vi "www template read file.vi"(6 "User Information":T1, 7 "HTTP Header (\"\")":string, 8 "error in (no error)":errorcluster, 11 "Template File (\"\")":string) -> (0 "error out":errorcluster, 3 "Page HTML":string, 5 "new HTTP Header":string)   [LabVIEW 2011]
uses:
  server/database/Users/User Record.ctl
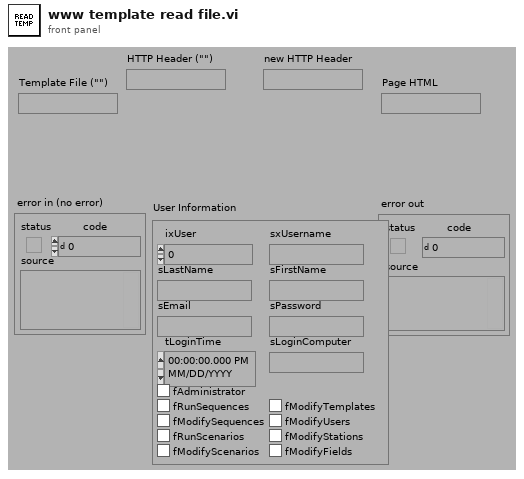
[diagram p1: front panel]
types:
  T1 = typedef "User Record.ctl" = cluster{"ixUser":i32, "sxUsername":string, "sLastName":string, "sFirstName":string, "sEmail":string, "sPassword":string, "tLoginTime":timestamp, "sLoginComputer":string, "fAdministrator":bool, "fRunSequences":bool, "fModifySequences":bool, "fRunScenarios":bool, "fModifyScenarios":bool, "fModifyTemplates":bool, "fModifyUsers":bool, "fModifyStations":bool, "fModifyFields":bool}
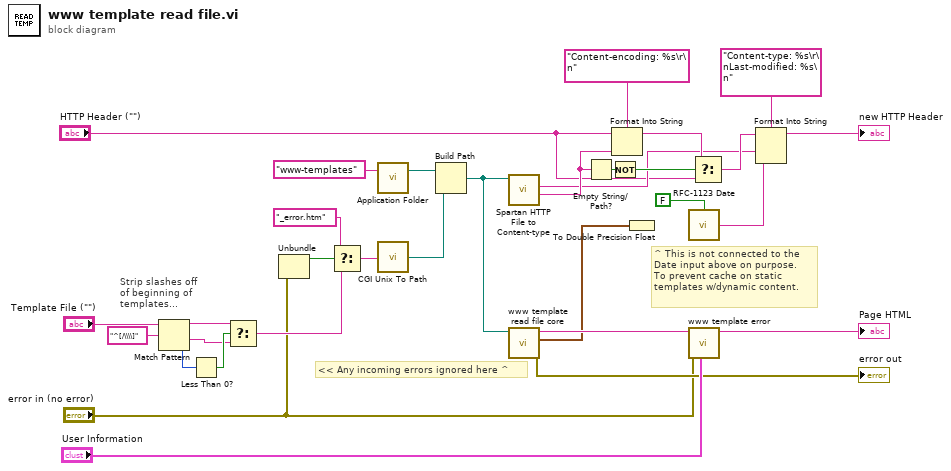
[diagram p0: block diagram]
diagram:
  # "Strip slashes off\nof beginning of\ntemplates..."
  # "^ This is not connected to the\nDate input above on purpose.\nTo prevent cache on static\ntemplates w/dynamic content."
  # "<< Any incoming errors ignored here ^"
  n1 = Match Pattern(string="Template File (\"\")", regular expression="^[/\\\\]") -> (before substring=w18:string, after substring=w17:string, offset past match=w20:i32)  [unwired: 2 out]
  n2 = Less Than 0?(x=w20) -> (x < 0?=w19:bool)
  n3 = Select(t=w18, s=w19, f=w17) -> (s? t:f=w9:string)
  n4 = Unbundle("error in (no error)") -> ("status"=w12:bool)  [unwired: 2 out]
  n5 = Select(t="_error.htm" ("format string"), s=w12, f=w9) -> (s? t:f=w10:string)
  n6 = call "Application Folder.vi"("Relative Path (\"\" - Folder)"="www-templates" ("name or relative path")) -> ("Application Folder"=w1:path)  [unwired: 2 in]
  n7 = call "CGI Unix To Path.vi"("unix path"=w10) -> ("platform path"=w22:path)  [unwired: 1 out]
  n8 = Build Path(base path=w1, name or relative path=w22) -> (appended path=w5:path)
  n9 = call "Spartan HTTP File to Content-type.vi"("file path"=w5) -> ("content-encoding"=w24:string, "content-type"=w23:string)  [unwired: 3 in, 6 out]
  n10 = call "www template read file core.vi"("Path"=w5) -> ("error out"=→"error out":errorcluster, "File Modified"=w3:timestamp, "File Content"=w6:string)  [unwired: 1 in, 7 out]
  n11 = Empty String/Path?(string/path=w24) -> (empty?=w29:bool)
  n12 = Not(x=w29) -> (.not. x?=w30:bool)
  n13 = Format Into String(format string="Content-encoding: %s\r\n", initial string="HTTP Header (\"\")", w24) -> (resulting string=w31:string)  [unwired: 1 in, 1 out]
  n14 = To Double Precision Float(number=w3) -> ()  [unwired: 1 out]
  n15 = call "RFC-1123 Date.vi"("numeric zone offset (true)"=FALSE) -> ("GMT Date/Time"=w26:string)  [unwired: 1 in]
  n16 = call "www template error.vi"("User Information"="User Information", "error in (no error)"="error in (no error)", "Incoming Template HTML (\"\")"=w6) -> ("error.htm"=→"Page HTML":string)  [unwired: 8 out]
  n17 = Select(t=w31, s=w30, f="HTTP Header (\"\")") -> (s? t:f=w32:string)
  n18 = Format Into String(format string="Content-type: %s\r\nLast-modified: %s\n" ("HTTP Header"), initial string=w32, w23, w26) -> (resulting string=→"new HTTP Header":string)  [unwired: 1 in, 1 out]
